vi "Parse Read Byte.vi"(0 "Read Byte":u8[](array[numeric]) format="%02x", 1 "FRU Information In":T1, 3 "error in (no error)":errorcluster, 4 "FRU Type":T2) -> (7 "FRU Information Out":T1, 10 "error out":errorcluster)   [LabVIEW 2016]
doc: "Get the FRU write array and its content (address byte and data byte) from CSV"
uses:
  Type Definitions/FRU Information.ctl
  Type Definitions/FRU Type.ctl
  SubVI/Conversion Type.ctl
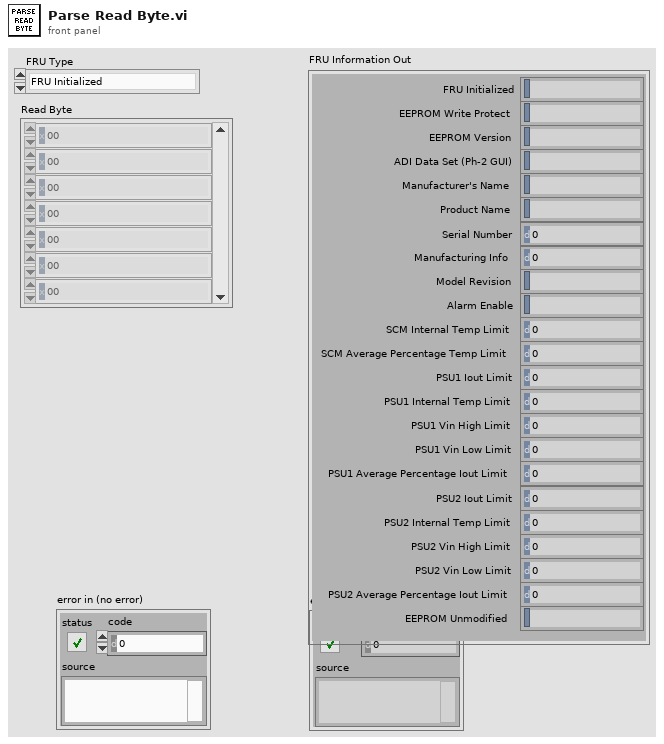
[diagram p1: front panel]
types:
  T1 = typedef "FRU Information.ctl" = cluster{"FRU Initialized":string, "EEPROM Write Protect":string, "EEPROM Version":string, "ADI Data Set (Ph-2 GUI)":string, "Manufacturer's Name":string, "Product Name":string, "Serial Number":u32, "Manufacturing Info":u32, "Model Revision":string, "Alarm Enable":string, "SCM Internal Temp Limit":u32, "SCM Average Percentage Temp Limit":u32, "PSU1 Iout Limit":u32, "PSU1 Internal Temp Limit":u32, "PSU1 Vin High Limit":u32, "PSU1 Vin Low Limit":u32, "PSU1 Average Percentage Iout Limit":u32, "PSU2 Iout Limit":u32, "PSU2 Internal Temp Limit":u32, "PSU2 Vin High Limit":u32, "PSU2 Vin Low Limit":u32, "PSU2 Average Percentage Iout Limit":u32, "EEPROM Unmodified":string}
  T2 = typedef "FRU Type.ctl" = enum16{"FRU Initialized", "EEROM Write Protect", "EEPROM Version", "ADI Data Set (Ph-2 GUI)", "Manufacturer's Name", "Product Name", "Serial Number", "Manufacturing Info", "Model Revision", "Alarm Enable", "SCM Internal Temp Limit", "SCM Average Percentage Temp Limit", "PSU1 Iout Limit", "PSU1 Internal Temp Limit", "PSU1 Vin High Limit", "PSU1 Vin Low Limit", "PSU1 Average Percentage Iout Limit", "PSU2 Iout Limit", "PSU2 Internal Temp Limit", "PSU2 Vin High Limit", "PSU2 Vin Low Limit", "PSU2 Average Percentage Iout Limit", "EEPROM Unmodified"}
  T3 = typedef "Conversion Type.ctl" = enum16{"String - ASCII", "String - HEX", "Numeric - DEC"}
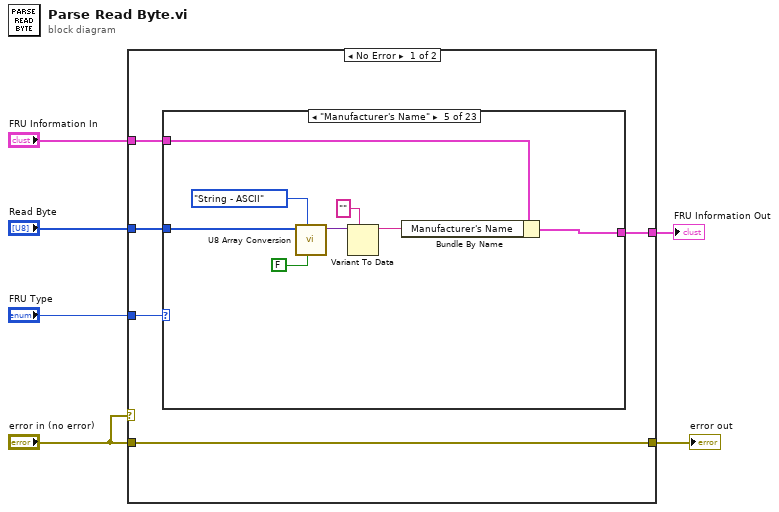
[diagram p0: block diagram]
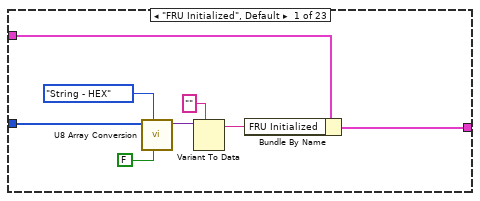
[diagram p2: hidden frame]
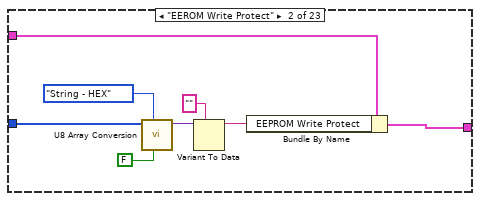
[diagram p3: hidden frame]
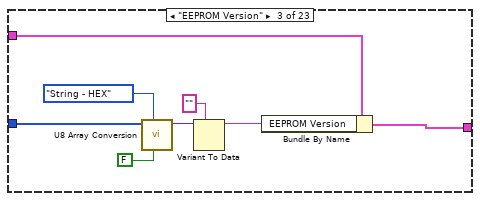
[diagram p4: hidden frame]
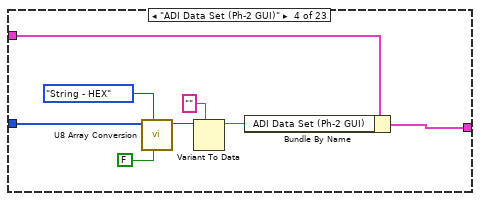
[diagram p5: hidden frame]
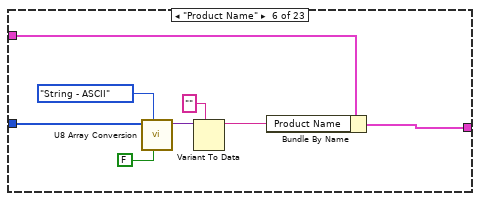
[diagram p6: hidden frame]
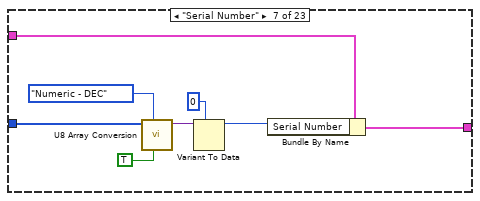
[diagram p7: hidden frame]
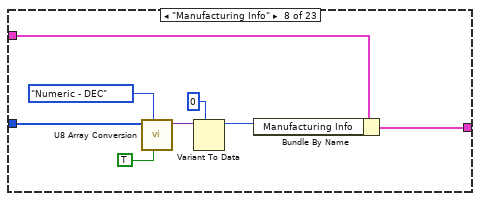
[diagram p8: hidden frame]
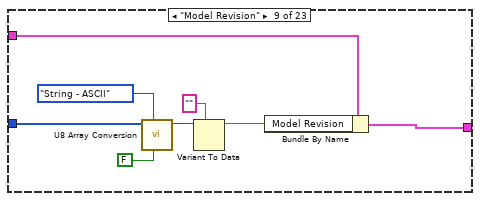
[diagram p9: hidden frame]
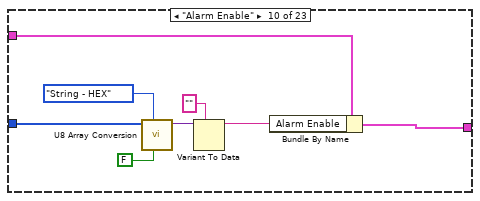
[diagram p10: hidden frame]
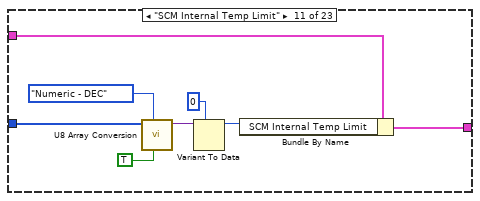
[diagram p11: hidden frame]
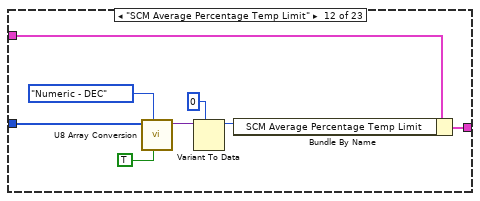
[diagram p12: hidden frame]
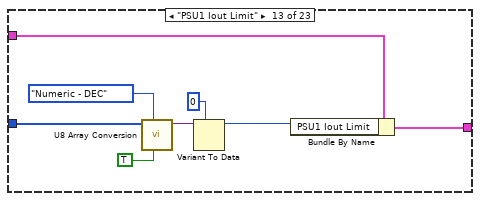
[diagram p13: hidden frame]
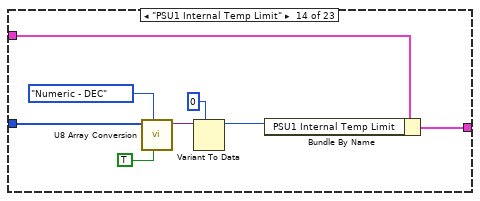
[diagram p14: hidden frame]
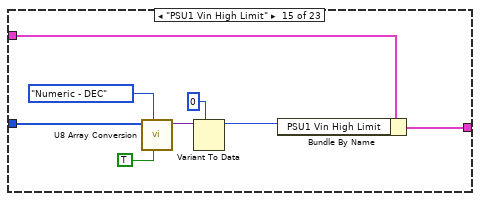
[diagram p15: hidden frame]
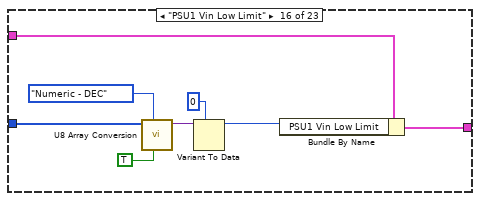
[diagram p16: hidden frame]
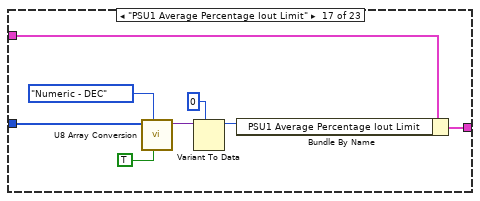
[diagram p17: hidden frame]
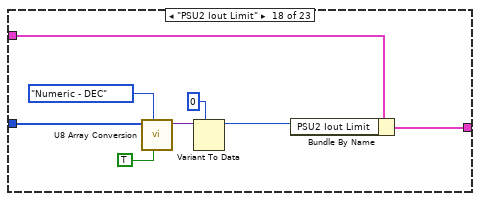
[diagram p18: hidden frame]
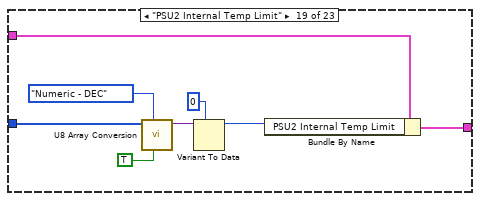
[diagram p19: hidden frame]
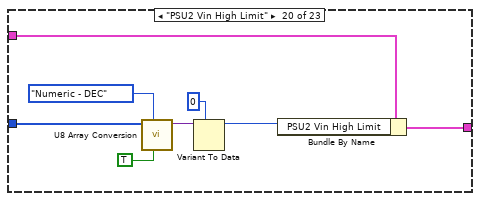
[diagram p20: hidden frame]
diagram:
  n1 = case shown="No Error" "error in (no error)" {
    tunnel: "FRU Type" -> [w10 _]
    tunnel: "error in (no error)" -> [w11 w197]
    tunnel: [w11 w197] -> w6
    tunnel: "Read Byte" -> [w9 _]
    tunnel: [w8 T1 {"FRU Initialized"="", "EEPROM Write Protect"="", "EEPROM Version"="", "ADI Data Set (Ph-2 GUI)"="", "Manufacturer's Name"="", "Product Name"="", "Serial Number"=0, "Manufacturing Info"=0, "Model Revision"="", "Alarm Enable"="", "SCM Internal Temp Limit"=0, "SCM Average Percentage Temp Limit"=0, "PSU1 Iout Limit"=0, "PSU1 Internal Temp Limit"=0, "PSU1 Vin High Limit"=0, "PSU1 Vin Low Limit"=0, "PSU1 Average Percentage Iout Limit"=0, "PSU2 Iout Limit"=0, "PSU2 Internal Temp Limit"=0, "PSU2 Vin High Limit"=0, "PSU2 Vin Low Limit"=0, "PSU2 Average Percentage Iout Limit"=0, "EEPROM Unmodified"=""} ("FRU Information")] -> w3
    tunnel: "FRU Information In" -> [w7 _]
    frame No Error {
      n2 = case shown="\"Manufacturer's Name\"" w10 {
        tunnel: w9 -> [w12 w20 w28 w36 w44 w52 w60 w68 w76 w85 w92 w100 w108 w116 w124 w132 w140 w148 w156 w164 w172 w180 w188]
        tunnel: [w17 w25 w33 w41 w49 w57 w65 w73 w81 w89 w97 w105 w113 w121 w129 w137 w145 w153 w161 w169 w177 w185 w193] -> w8
        tunnel: w7 -> [w14 w22 w30 w38 w46 w55 w64 w72 w79 w87 w96 w104 w112 w120 w128 w136 w144 w152 w160 w168 w176 w184 w190]
        frame "FRU Initialized", Default {
          n3 = call "U8 Array Conversion.vi"("Reverse"=FALSE, "Conversion Type"=Conversion_Type."String - HEX", "U8 Array"=w12) -> ("Conversion Output"=w18:variant)  [unwired: 8 in]
          n4 = Variant To Data(type="", Variant=w18) -> (data=w16:string)  [unwired: 1 in, 1 out]
          n5 = Bundle By Name(cluster=w14, "FRU Initialized"=w16) -> (w17:T1)
        }
        frame "EEROM Write Protect" {
          n6 = call "U8 Array Conversion.vi"("Reverse"=FALSE, "Conversion Type"=Conversion_Type."String - HEX", "U8 Array"=w20) -> ("Conversion Output"=w26:variant)  [unwired: 8 in]
          n7 = Variant To Data(type="", Variant=w26) -> (data=w24:string)  [unwired: 1 in, 1 out]
          n8 = Bundle By Name(cluster=w22, "EEPROM Write Protect"=w24) -> (w25:T1)
        }
        frame "EEPROM Version" {
          n9 = call "U8 Array Conversion.vi"("Reverse"=FALSE, "Conversion Type"=Conversion_Type."String - HEX", "U8 Array"=w28) -> ("Conversion Output"=w34:variant)  [unwired: 8 in]
          n10 = Variant To Data(type="", Variant=w34) -> (data=w32:string)  [unwired: 1 in, 1 out]
          n11 = Bundle By Name(cluster=w30, "EEPROM Version"=w32) -> (w33:T1)
        }
        frame "ADI Data Set (Ph-2 GUI)" {
          n12 = call "U8 Array Conversion.vi"("Reverse"=FALSE, "Conversion Type"=Conversion_Type."String - HEX", "U8 Array"=w36) -> ("Conversion Output"=w42:variant)  [unwired: 8 in]
          n13 = Variant To Data(type="", Variant=w42) -> (data=w40:string)  [unwired: 1 in, 1 out]
          n14 = Bundle By Name(cluster=w38, "ADI Data Set (Ph-2 GUI)"=w40) -> (w41:T1)
        }
        frame "Manufacturer's Name" {
          n15 = call "U8 Array Conversion.vi"("Reverse"=FALSE, "Conversion Type"=Conversion_Type."String - ASCII", "U8 Array"=w44) -> ("Conversion Output"=w50:variant)  [unwired: 8 in]
          n16 = Variant To Data(type="", Variant=w50) -> (data=w48:string)  [unwired: 1 in, 1 out]
          n17 = Bundle By Name(cluster=w46, "Manufacturer's Name"=w48) -> (w49:T1)
        }
        frame "Product Name" {
          n18 = call "U8 Array Conversion.vi"("Reverse"=FALSE, "Conversion Type"=Conversion_Type."String - ASCII", "U8 Array"=w52) -> ("Conversion Output"=w58:variant)  [unwired: 8 in]
          n19 = Variant To Data(type="", Variant=w58) -> (data=w54:string)  [unwired: 1 in, 1 out]
          n20 = Bundle By Name(cluster=w55, "Product Name"=w54) -> (w57:T1)
        }
        frame "Serial Number" {
          n21 = call "U8 Array Conversion.vi"("Reverse"=TRUE, "Conversion Type"=Conversion_Type."Numeric - DEC", "U8 Array"=w60) -> ("Conversion Output"=w66:variant)  [unwired: 8 in]
          n22 = Variant To Data(type=u32 0 ("Serial Number"), Variant=w66) -> (data=w62:u32)  [unwired: 1 in, 1 out]
          n23 = Bundle By Name(cluster=w64, "Serial Number"=w62) -> (w65:T1)
        }
        frame "Manufacturing Info" {
          n24 = call "U8 Array Conversion.vi"("Reverse"=TRUE, "Conversion Type"=Conversion_Type."Numeric - DEC", "U8 Array"=w68) -> ("Conversion Output"=w74:variant)  [unwired: 8 in]
          n25 = Variant To Data(type=u32 0 ("Serial Number"), Variant=w74) -> (data=w70:u32)  [unwired: 1 in, 1 out]
          n26 = Bundle By Name(cluster=w72, "Manufacturing Info"=w70) -> (w73:T1)
        }
        frame "Model Revision" {
          n27 = call "U8 Array Conversion.vi"("Reverse"=FALSE, "Conversion Type"=Conversion_Type."String - ASCII", "U8 Array"=w76) -> ("Conversion Output"=w82:variant)  [unwired: 8 in]
          n28 = Variant To Data(type="", Variant=w82) -> (data=w78:string)  [unwired: 1 in, 1 out]
          n29 = Bundle By Name(cluster=w79, "Model Revision"=w78) -> (w81:T1)
        }
        frame "Alarm Enable" {
          n30 = call "U8 Array Conversion.vi"("Reverse"=FALSE, "Conversion Type"=Conversion_Type."String - HEX", "U8 Array"=w85) -> ("Conversion Output"=w90:variant)  [unwired: 8 in]
          n31 = Variant To Data(type="", Variant=w90) -> (data=w86:string)  [unwired: 1 in, 1 out]
          n32 = Bundle By Name(cluster=w87, "Alarm Enable"=w86) -> (w89:T1)
        }
        frame "SCM Internal Temp Limit" {
          n33 = call "U8 Array Conversion.vi"("Reverse"=TRUE, "Conversion Type"=Conversion_Type."Numeric - DEC", "U8 Array"=w92) -> ("Conversion Output"=w98:variant)  [unwired: 8 in]
          n34 = Variant To Data(type=u32 0 ("Serial Number"), Variant=w98) -> (data=w94:u32)  [unwired: 1 in, 1 out]
          n35 = Bundle By Name(cluster=w96, "SCM Internal Temp Limit"=w94) -> (w97:T1)
        }
        frame "SCM Average Percentage Temp Limit" {
          n36 = call "U8 Array Conversion.vi"("Reverse"=TRUE, "Conversion Type"=Conversion_Type."Numeric - DEC", "U8 Array"=w100) -> ("Conversion Output"=w106:variant)  [unwired: 8 in]
          n37 = Variant To Data(type=u32 0 ("Serial Number"), Variant=w106) -> (data=w102:u32)  [unwired: 1 in, 1 out]
          n38 = Bundle By Name(cluster=w104, "SCM Average Percentage Temp Limit"=w102) -> (w105:T1)
        }
        frame "PSU1 Iout Limit" {
          n39 = call "U8 Array Conversion.vi"("Reverse"=TRUE, "Conversion Type"=Conversion_Type."Numeric - DEC", "U8 Array"=w108) -> ("Conversion Output"=w114:variant)  [unwired: 8 in]
          n40 = Variant To Data(type=u32 0 ("Serial Number"), Variant=w114) -> (data=w110:u32)  [unwired: 1 in, 1 out]
          n41 = Bundle By Name(cluster=w112, "PSU1 Iout Limit"=w110) -> (w113:T1)
        }
        frame "PSU1 Internal Temp Limit" {
          n42 = call "U8 Array Conversion.vi"("Reverse"=TRUE, "Conversion Type"=Conversion_Type."Numeric - DEC", "U8 Array"=w116) -> ("Conversion Output"=w122:variant)  [unwired: 8 in]
          n43 = Variant To Data(type=u32 0 ("Serial Number"), Variant=w122) -> (data=w118:u32)  [unwired: 1 in, 1 out]
          n44 = Bundle By Name(cluster=w120, "PSU1 Internal Temp Limit"=w118) -> (w121:T1)
        }
        frame "PSU1 Vin High Limit" {
          n45 = call "U8 Array Conversion.vi"("Reverse"=TRUE, "Conversion Type"=Conversion_Type."Numeric - DEC", "U8 Array"=w124) -> ("Conversion Output"=w130:variant)  [unwired: 8 in]
          n46 = Variant To Data(type=u32 0 ("Serial Number"), Variant=w130) -> (data=w126:u32)  [unwired: 1 in, 1 out]
          n47 = Bundle By Name(cluster=w128, "PSU1 Vin High Limit"=w126) -> (w129:T1)
        }
        frame "PSU1 Vin Low Limit" {
          n48 = call "U8 Array Conversion.vi"("Reverse"=TRUE, "Conversion Type"=Conversion_Type."Numeric - DEC", "U8 Array"=w132) -> ("Conversion Output"=w138:variant)  [unwired: 8 in]
          n49 = Variant To Data(type=u32 0 ("Serial Number"), Variant=w138) -> (data=w134:u32)  [unwired: 1 in, 1 out]
          n50 = Bundle By Name(cluster=w136, "PSU1 Vin Low Limit"=w134) -> (w137:T1)
        }
        frame "PSU1 Average Percentage Iout Limit" {
          n51 = call "U8 Array Conversion.vi"("Reverse"=TRUE, "Conversion Type"=Conversion_Type."Numeric - DEC", "U8 Array"=w140) -> ("Conversion Output"=w146:variant)  [unwired: 8 in]
          n52 = Variant To Data(type=u32 0 ("Serial Number"), Variant=w146) -> (data=w142:u32)  [unwired: 1 in, 1 out]
          n53 = Bundle By Name(cluster=w144, "PSU1 Average Percentage Iout Limit"=w142) -> (w145:T1)
        }
        frame "PSU2 Iout Limit" {
          n54 = call "U8 Array Conversion.vi"("Reverse"=TRUE, "Conversion Type"=Conversion_Type."Numeric - DEC", "U8 Array"=w148) -> ("Conversion Output"=w154:variant)  [unwired: 8 in]
          n55 = Variant To Data(type=u32 0 ("Serial Number"), Variant=w154) -> (data=w150:u32)  [unwired: 1 in, 1 out]
          n56 = Bundle By Name(cluster=w152, "PSU2 Iout Limit"=w150) -> (w153:T1)
        }
        frame "PSU2 Internal Temp Limit" {
          n57 = call "U8 Array Conversion.vi"("Reverse"=TRUE, "Conversion Type"=Conversion_Type."Numeric - DEC", "U8 Array"=w156) -> ("Conversion Output"=w162:variant)  [unwired: 8 in]
          n58 = Variant To Data(type=u32 0 ("Serial Number"), Variant=w162) -> (data=w158:u32)  [unwired: 1 in, 1 out]
          n59 = Bundle By Name(cluster=w160, "PSU2 Internal Temp Limit"=w158) -> (w161:T1)
        }
        frame "PSU2 Vin High Limit" {
          n60 = call "U8 Array Conversion.vi"("Reverse"=TRUE, "Conversion Type"=Conversion_Type."Numeric - DEC", "U8 Array"=w164) -> ("Conversion Output"=w170:variant)  [unwired: 8 in]
          n61 = Variant To Data(type=u32 0 ("Serial Number"), Variant=w170) -> (data=w166:u32)  [unwired: 1 in, 1 out]
          n62 = Bundle By Name(cluster=w168, "PSU2 Vin High Limit"=w166) -> (w169:T1)
        }
        frame "PSU2 Vin Low Limit" {
          n63 = call "U8 Array Conversion.vi"("Reverse"=TRUE, "Conversion Type"=Conversion_Type."Numeric - DEC", "U8 Array"=w172) -> ("Conversion Output"=w178:variant)  [unwired: 8 in]
          n64 = Variant To Data(type=u32 0 ("Serial Number"), Variant=w178) -> (data=w174:u32)  [unwired: 1 in, 1 out]
          n65 = Bundle By Name(cluster=w176, "PSU2 Vin Low Limit"=w174) -> (w177:T1)
        }
        frame "PSU2 Average Percentage Iout Limit" {
          n66 = call "U8 Array Conversion.vi"("Reverse"=TRUE, "Conversion Type"=Conversion_Type."Numeric - DEC", "U8 Array"=w180) -> ("Conversion Output"=w186:variant)  [unwired: 8 in]
          n67 = Variant To Data(type=u32 0 ("Serial Number"), Variant=w186) -> (data=w182:u32)  [unwired: 1 in, 1 out]
          n68 = Bundle By Name(cluster=w184, "PSU2 Average Percentage Iout Limit"=w182) -> (w185:T1)
        }
        frame "EEPROM Unmodified" {
          n69 = call "U8 Array Conversion.vi"("Reverse"=FALSE, "Conversion Type"=Conversion_Type."String - HEX", "U8 Array"=w188) -> ("Conversion Output"=w194:variant)  [unwired: 8 in]
          n70 = Variant To Data(type="", Variant=w194) -> (data=w192:string)  [unwired: 1 in, 1 out]
          n71 = Bundle By Name(cluster=w190, "EEPROM Unmodified"=w192) -> (w193:T1)
        }
      }
    }
    frame Error {
    }
  }
  "error out" <- w6
  "FRU Information Out" <- w3
